vi "Default_TestMode_40KHZ.vi"() -> ()   [LabVIEW 2017]
panel:
  out "Test Result":picture
  out "XY Graph":cluster{dbl, u32}[](graph)
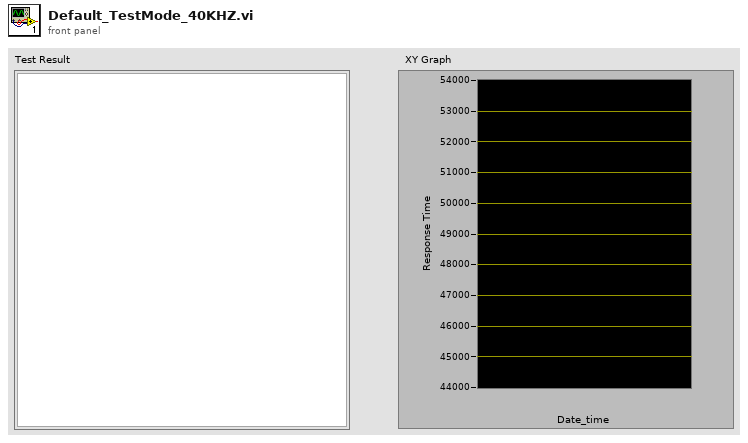
[diagram p1: front panel]
types:
  T1 = enum16{"open", "replace", "create", "open or create", "replace or create", "replace or create with confirmation"}
  T2 = cluster{"[0]":string, "[1]":string, "[2]":string, "[3]":string, "[4]":string, "[5]":string, "[6]":string, "[7]":string, "[8]":string}
  T3 = cluster{"Iterations":u64, "DelayBetweenIterations":u32, "Timeout":u32, "MessageID":i32, "MessageLength":i32, "ResponseID":i32, "Timestamp":string, "TestSuite":string, "ReportPath":path, "FWVersionPath":path}
  T4 = cluster{"Socket_IP_Address":string, "Socket_Port_Number":u16, "Global_ReportPath":path}
  T5 = typedef "imagedata.ctl" = cluster{"image type":i32, "image depth":i32, "image":u8[], "mask":u8[], "colors":u32[], "Rectangle":cluster{"left":i16, "top":i16, "right":i16, "bottom":i16}}
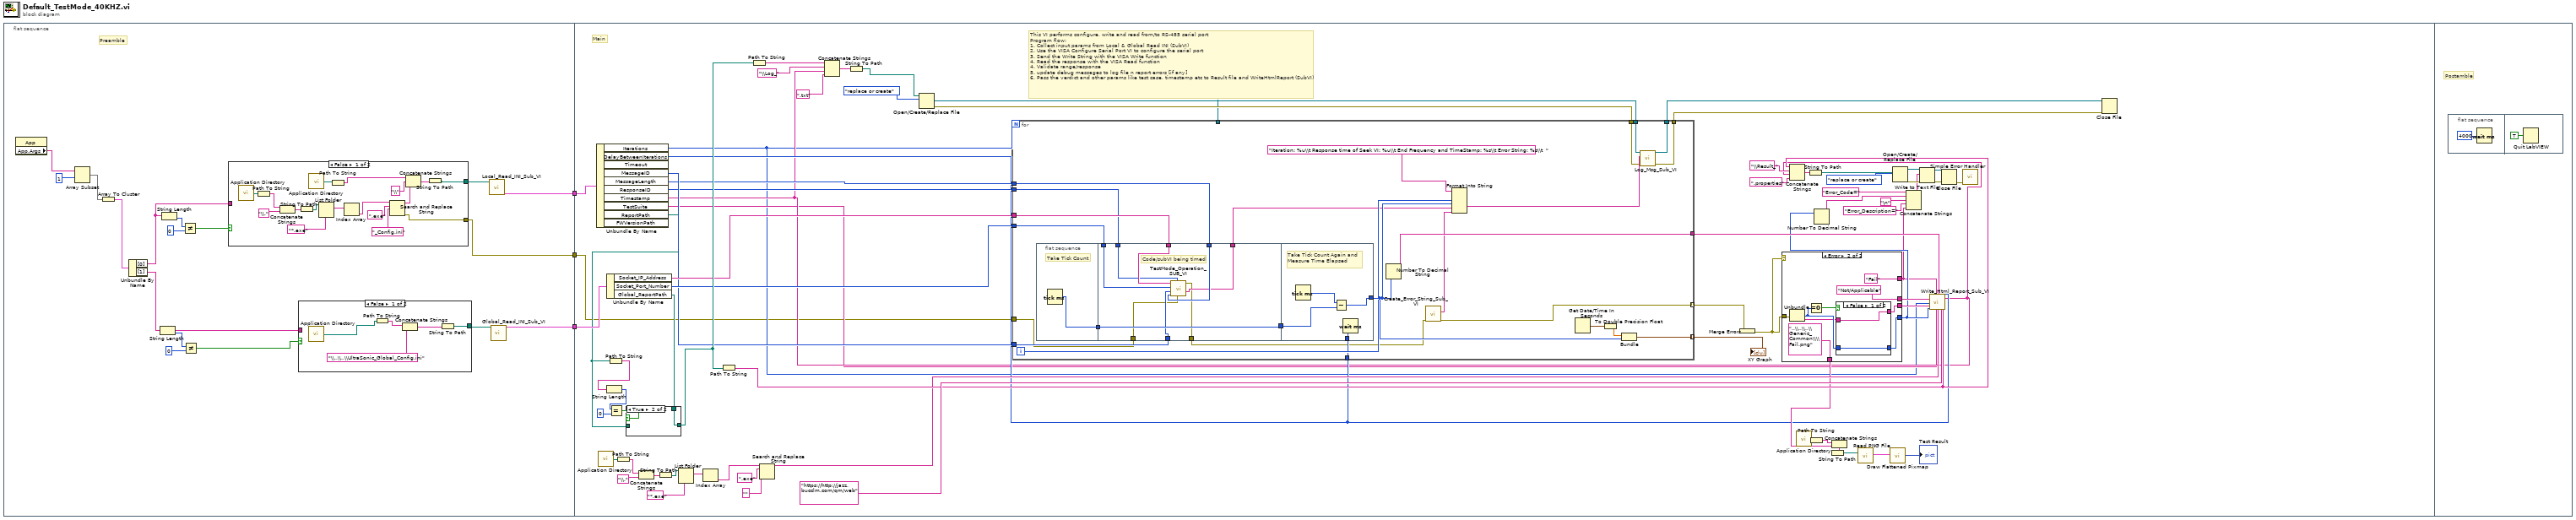
[diagram p0: block diagram]
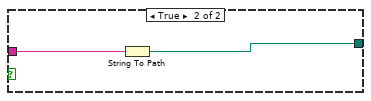
[diagram p2: hidden frame]
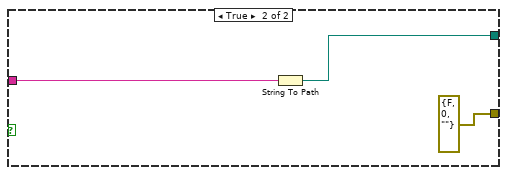
[diagram p3: hidden frame]
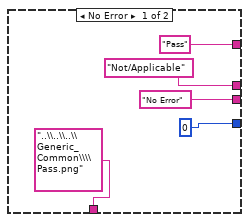
[diagram p5: hidden frame]
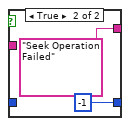
[diagram p6: hidden frame]
diagram:
  n1 = flat-sequence {
    tunnel: [w6] -> w3
    tunnel: [w5] -> w2
    tunnel: [w4] -> w1
    tunnel: w3 -> [w48]
    tunnel: w2 -> [w62]
    tunnel: w1 -> [w58]
    frame #0 {
      # "Preamble"
      n2 = property class="App"() -> ("App.Args"=w8:string[])  [unwired: 2 in, 2 out]
      n3 = Array Subset "Array Subset"(array=w8, index=1) -> (w9:string[])  [unwired: 1 in]
      n4 = Array To Cluster(array=w9) -> (cluster=w10:T2)
      n5 = Unbundle By Name "Unbundle By Name"(w10) -> ("[0]"=w14:string, "[1]"=w17:string)
      n6 = String Length(string=w17) -> (length=w18:i32)
      n7 = String Length(string=w14) -> (length=w11:i32)
      n8 = Not Equal?(x=w11, y=0) -> (x != y?=w13:bool)
      n9 = Not Equal?(x=w18, y=0) -> (x != y?=w16:bool)
      n10 = case shown="False" w13 {
        tunnel: w14 -> [_ w47]
        tunnel: [w29 w46] -> w19
        tunnel: [w28 errorcluster {"status"=FALSE, "code"=0, "source"=""} ("error out")] -> w6
        frame False {
          n11 = call <vilib>:"Application Directory.vi"() -> ("Application Directory"=w35:path)
          n12 = Path To String(path=w35) -> (string=w34:string)
          n13 = Concatenate Strings(w34, "\\." ("string")) -> (w32:string)
          n14 = String To Path(string=w32) -> (path=w37:path)
          n15 = call <vilib>:"Application Directory.vi"() -> ("Application Directory"=w44:path)
          n16 = List Folder(path=w37, pattern="*.exe") -> (filenames=w31:string[])  [unwired: 2 in, 3 out]
          n17 = Path To String(path=w44) -> (string=w39:string)
          n18 = Index Array(array=w31) -> (element=w30:string)  [unwired: 1 in]
          n19 = Search and Replace String(input string=w30, search string=".exe", replace string="_Config.ini" ("replace string (\"\")")) -> (result string=w41:string, error out=w28:errorcluster)  [unwired: 5 in, 2 out]
          n20 = Concatenate Strings(w39, "\\" ("string"), w41) -> (w38:string)
          n21 = String To Path(string=w38) -> (path=w29:path)
        }
        frame True {
          n22 = String To Path(string=w47) -> (path=w46:path)
        }
      }
      n23 = case shown="False" w16 {
        tunnel: [w22 w27] -> w20
        tunnel: w17 -> [_ w26]
        frame False {
          n24 = call <vilib>:"Application Directory.vi"() -> ("Application Directory"=w21:path)
          n25 = Path To String(path=w21) -> (string=w25:string)
          n26 = Concatenate Strings(w25, "\\..\\..\\UltraSonic_Global_Config.ini" ("string")) -> (w23:string)
          n27 = String To Path(string=w23) -> (path=w22:path)
        }
        frame True {
          n28 = String To Path(string=w26) -> (path=w27:path)
        }
      }
      n29 = call "Local_Read_INI_Sub_VI.vi"("Config File Path"=w19) -> ("output cluster"=w4:T3)  [unwired: 10 in]
      n30 = call "Global_Read_INI_Sub_VI.vi"("Config File Path"=w20) -> ("output cluster"=w5:T4)  [unwired: 14 in]
    }
    frame #1 {
      # "This VI performs configure, write and read from/to RS-485 serial port\nProgram flow:\n1. Collect input params from Local & Global Read INI (SubVI)\n2. Use the VISA Configure Serial Port VI to configure the serial port\n3. Send the Write String with the VISA Write function\n4. Read the response with the VISA Read function\n4. Validate range/response\n5. update debug messages to log file n report errors [if any]\n6. Pass the verdict and other params like test case, timestamp etc to Result file and WriteHtmlReport (SubVI)"
      # "Main"
      n31 = Unbundle By Name(w58) -> ("Iterations"=w50:u64, "DelayBetweenIterations"=w54:u32, "MessageID"=w57:i32, "MessageLength"=w56:i32, "ResponseID"=w55:i32, "Timestamp"=w52:string, "TestSuite"=w51:string, "ReportPath"=w49:path)  [unwired: 2 out]
      n32 = call <vilib>:"Application Directory.vi"() -> ("Application Directory"=w78:path)
      n33 = Unbundle By Name(w62) -> ("Socket_IP_Address"=w60:string, "Socket_Port_Number"=w59:u16, "Global_ReportPath"=w61:path)
      n34 = Path To String(path=w49) -> (string=w109:string)
      n35 = String Length(string=w109) -> (length=w108:i32)
      n36 = Equal?(x=w108, y=0) -> (x = y?=w106:bool)
      n37 = Path To String(path=w78) -> (string=w77:string)
      n38 = case shown="True" w106 {
        tunnel: w61 -> [_ w121]
        tunnel: [w120 w121] -> w105
        tunnel: w49 -> [w120 _]
        frame False {
        }
        frame True {
        }
      }
      n39 = Concatenate Strings(w77, "\\." ("string")) -> (w75:string)
      n40 = String To Path(string=w75) -> (path=w80:path)
      n41 = List Folder(path=w80, pattern="*.exe") -> (filenames=w74:string[])  [unwired: 2 in, 3 out]
      n42 = Index Array(array=w74) -> (element=w70:string)  [unwired: 1 in]
      n43 = Path To String(path=w105) -> (string=w82:string)
      n44 = Path To String(path=w105) -> (string=w111:string)
      n45 = Search and Replace String(input string=w70, search string=".exe", replace string="" ("replace string (\"\")")) -> (result string=w73:string)  [unwired: 5 in, 3 out]
      n46 = Concatenate Strings(w111, "\\Log_" ("string"), w52, ".txt" ("string")) -> (w114:string)
      n47 = String To Path(string=w114) -> (path=w113:path)
      n48 = Open/Create/Replace File(file path (use dialog)=w113, operation (0:open)=T1."replace or create") -> (refnum out=w83:refnum<file>, error out=w86:errorcluster)  [unwired: 1 in, 4 out]
      n49 = for {
        N: w50 -> [_]
        tunnel: [w144] -> w117
        tunnel: w83 -> [w138]
        tunnel: [w137] -> w85
        tunnel: [w135] -> w84
        tunnel: [w140] -> w115 mode=indexing
        tunnel: w86 -> [w136]
        tunnel: w83 -> [_]
        tunnel: [w132] -> w81 mode=indexing
        tunnel: w60 -> [w131]
        tunnel: w59 -> [w130]
        tunnel: w57 -> [w129]
        tunnel: w56 -> [w128]
        tunnel: w55 -> [w125]
        tunnel: w54 -> [w127]
        tunnel: w48 -> [w124]
        i -> [w133]
        n50 = flat-sequence {
          tunnel: [w147] -> w146
          tunnel: [w156] -> w145
          tunnel: w146 -> [w156]
          tunnel: w131 -> [w155]
          tunnel: w130 -> [w154]
          tunnel: w129 -> [w153]
          tunnel: w128 -> [w152]
          tunnel: w125 -> [w151]
          tunnel: w124 -> [w150]
          tunnel: [w149] -> w123
          tunnel: [w148] -> w122
          tunnel: w145 -> [w160]
          tunnel: [w158] -> w134
          tunnel: w127 -> [w157]
          frame #0 {
            # "Take Tick Count"
            n51 = Tick Count (ms)() -> (millisecond timer value=w147:u32)
          }
          frame #1 {
            # "Code/subVI being timed"
            n52 = call "TestMode_Operation_SUB_VI.vi"("error in (no error)"=w150, "Response ID 1"=w151, "Operation Message Length 1"=w152, "Operation Message ID 1"=w153, "Socket Port"=w154, "Socket IP Adress"=w155) -> ("End frequency and Time Stamp 2"=w149:string, "error out"=w148:errorcluster)  [unwired: 4 in]
          }
          frame #2 {
            # "Take Tick Count Again and Measure Time Elapsed"
            n53 = Tick Count (ms)() -> (millisecond timer value=w159:u32)
            n54 = Subtract(x=w159, y=w160) -> (x-y=w158:u32)
            n55 = Wait (ms)(milliseconds to wait=w157) -> ()  [unwired: 1 out]
          }
        }
        n56 = Number To Decimal String(number=w134) -> (decimal integer string=w144:string)  [unwired: 1 in]
        n57 = call "Create_Error_String_Sub_VI.vi"("error in"=w122) -> ("error out"=w132:errorcluster, "Error String"=w126:string)  [unwired: 9 in]
        n58 = Format Into String(format string="Iteration: %u\\t Response time of Seek VI: %u\\t End Frequency and TimeStamp: %s\\t Error String: %s\\t  ", w133, w134, w123, w126) -> (resulting string=w139:string)  [unwired: 2 in, 1 out]
        n59 = Get Date/Time In Seconds() -> (seconds since 1Jan1904=w141:timestamp)
        n60 = To Double Precision Float(number=w141) -> (double precision float=w142:dbl)
        n61 = Bundle "Bundle"(w142, w134) -> (w140:cluster{dbl, u32})  [unwired: 1 in]
        n62 = call "Log_Msg_Sub_VI.vi"("error in (no error)"=w136, "String"=w139, "Byte Stream File in"=w138) -> ("error out"=w135:errorcluster, "Byte Stream File out"=w137:refnum<file>)  [unwired: 7 in]
      }
      "XY Graph" <- w115
      n63 = Merge Errors "Merge Errors"(w81) -> (w53:errorcluster)
      n64 = case shown="Error" w53 {
        tunnel: ["Pass" "Fail"] -> w87
        tunnel: w53 -> [_ w172]
        tunnel: [0 ("code") w168] -> w91
        tunnel: ["No Error" ("source") w169] -> w119
        tunnel: ["Not/Applicable" "Not/Applicable"] -> w118
        tunnel: ["..\\..\\..\\Generic_Common\\\\Pass.png" ("string") "..\\..\\..\\Generic_Common\\\\Fail.png" ("string")] -> w63
        frame No Error {
        }
        frame Error {
          n65 = Unbundle(w172) -> ("code"=w170:i32, "source"=w166:string)  [unwired: 1 out]
          n66 = Equal To 0?(x=w170) -> (x = 0?=w167:bool)
          n67 = case shown="False" w167 {
            tunnel: [w176 -1 ("code")] -> w168
            tunnel: [w175 "Seek Operation Failed" ("source")] -> w169
            tunnel: w170 -> [w176 _]
            tunnel: w166 -> [w175 _]
            frame False {
            }
            frame True {
            }
          }
        }
      }
      n68 = Concatenate Strings(w82, "\\Result_" ("string"), w52, ".properties" ("string")) -> (w103:string)
      n69 = call <vilib>:"Application Directory.vi"() -> ("Application Directory"=w64:path)
      n70 = String To Path(string=w103) -> (path=w95:path)
      n71 = Path To String(path=w64) -> (string=w65:string)
      n72 = Number To Decimal String(number=w91) -> (decimal integer string=w90:string)  [unwired: 1 in]
      n73 = Concatenate Strings(w65, w63) -> (w66:string)
      n74 = String To Path(string=w66) -> (path=w69:path)
      n75 = call <vilib>:"Read PNG File.vi"("path to PNG file"=w69) -> ("image data"=w67:T5)  [unwired: 8 in, 2 out]
      n76 = call <vilib>:"Draw Flattened Pixmap.vi"("image data"=w67) -> ("new picture"=→"Test Result":picture)  [unwired: 8 in]
      n77 = Open/Create/Replace File(file path (use dialog)=w95, operation (0:open)=T1."replace or create") -> (refnum out=w94:refnum<file>, error out=w99:errorcluster)  [unwired: 4 in, 1 out]
      n78 = Concatenate Strings("Error_Code=" ("string"), w90, "\n", "Error_Description=" ("string"), w87) -> (w93:string)
      n79 = Write to Text File(file (use dialog)=w94, text=w93, error in=w99) -> (refnum out=w98:refnum<file>, error out=w97:errorcluster)  [unwired: 1 in, 1 out]
      n80 = call "Write_Html_Report_Sub_VI.vi"("ReprtPath"=w82, "Remarks"=w118, "Iterations"=w50, "Error Description"=w119, "Timestamp"=w52, "TestCase"=w73, "Verdict"=w87, "TestSuite"=w51, "Time taken to execute  test in msec"=w117, "JazzDashboardLink"="https://http://jazz.bucclm.com/qm/web" ("TestSuite"), "Delay Between Iterations"=w54, "Error Code"=w91) -> ()  [unwired: 8 in]
      n81 = Close File(refnum=w98, error in=w97) -> (error out=w96:errorcluster)  [unwired: 1 out]
      n82 = call <vilib>:"Simple Error Handler.vi"("error in (no error)"=w96) -> ()  [unwired: 4 in, 5 out]
      n83 = Close File(refnum=w85, error in=w84) -> ()  [unwired: 2 out]
    }
    frame #2 {
      # "Postamble"
      n84 = flat-sequence {
        frame #0 {
          n85 = Wait (ms)(milliseconds to wait=u32 4000) -> ()  [unwired: 1 out]
        }
        frame #1 {
          n86 = Quit LabVIEW(quit? (T)=TRUE) -> ()
        }
      }
    }
  }
